vi "create_MagFieldTableObjects.vi"(8 "error in (no error)":errorcluster) -> (0 "error out":errorcluster)   [LabVIEW 2017]
doc: "loads the magfield table data from the MagFieldTables.ini and creates all MagfieldTable objects"
uses:
  Classes/MagFieldTable/MagFieldTable.lvclass
  global variables.vi
  <vilib>/Utility/config.llb/Read Key (String).vi
  Classes/StatusLog/StatusLog.lvclass
  <vilib>/Utility/config.llb/NI_LVConfig.lvlib
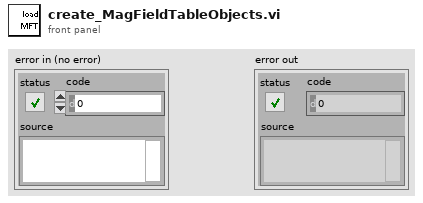
[diagram p1: front panel]
types:
  T1 = typedef "NI_LVConfig.lvlib/Config Data RefNum.ctl" = refnum<k1>
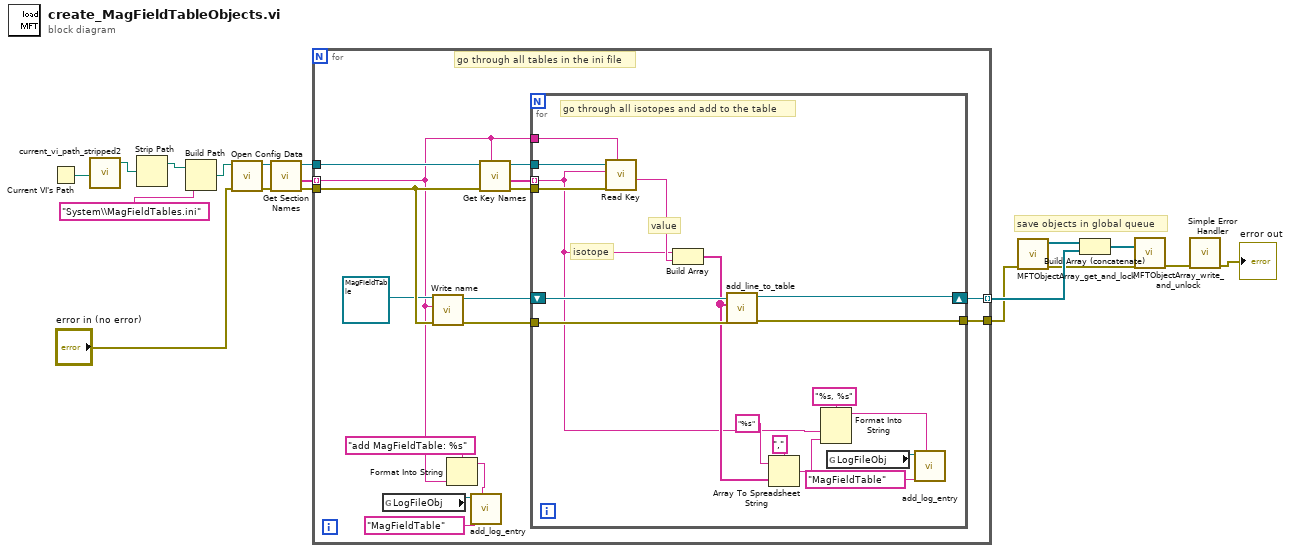
[diagram p0: block diagram]
diagram:
  # "save objects in global queue"
  n1 = Current VI's Path() -> (path=w14:path)
  n2 = call "current_vi_path_stripped2.vi"("current VI Path"=w14) -> ("current VI Path stripped out"=w12:path)  [unwired: 3 in, 1 out]
  n3 = Strip Path(path=w12) -> (stripped path=w13:path)  [unwired: 1 out]
  n4 = Build Path(base path=w13, name or relative path="System\\MagFieldTables.ini") -> (appended path=w15:path)
  n5 = call <vilib>:"Open Config Data.vi"("error in (no error)"="error in (no error)", "configuration file path"=w15) -> ("error out"=w16:errorcluster, "refnum"=w17:T1)  [unwired: 7 in, 1 out]
  n6 = call <vilib>:"Get Section Names.vi"("error in (no error)"=w16, "refnum"=w17) -> ("error out"=w9:errorcluster, "section names"=w11:string[], "refnum out"=w10:T1)  [unwired: 7 in]
  n7 = for {
    tunnel: w11 -> [w20] mode=indexing
    tunnel: w10 -> [w33]
    tunnel: w9 -> [w32]
    tunnel: [w25] -> w5 mode=indexing
    tunnel: [w24] -> w4
    # "go through all tables in the ini file"
    n8 = global read "global variables.vi" "LogFileObj"() -> (w23:refnum<class "StatusLog.lvclass">)
    n9 = call-dynamic "Write name.vi"("error in (no error)"=w32, "name"=w20, "MagFieldTable in"=refnum<class "MagFieldTable.lvclass"> refnum ("MagFieldTable.lvclass")) -> ("error out"=w27:errorcluster, "MagFieldTable out"=w28:refnum<class "MagFieldTable.lvclass">)  [unwired: 7 in]
    n10 = Format Into String(format string="add MagFieldTable: %s", w20) -> (resulting string=w19:string)  [unwired: 2 in, 1 out]
    n11 = call-dynamic "add_log_entry.vi"("new entry"=w19, "log identifiers"="MagFieldTable", "StatusLog in"=w23) -> ()  [unwired: 5 in, 2 out]
    n12 = call <vilib>:"Get Key Names.vi"("section"=w20, "error in (no error)"=w32, "refnum"=w33) -> ("error out"=w30:errorcluster, "key names"=w29:string[], "refnum out"=w31:T1)  [unwired: 5 in, 1 out]
    n13 = for {
      tunnel: w31 -> [w50]
      tunnel: w30 -> [w49]
      tunnel: w29 -> [w35] mode=indexing
      shift-right: [w44] -> w25
      shift-left: w28 -> [w46]
      tunnel: w27 -> [w45]
      tunnel: w20 -> [w48]
      tunnel: [w43] -> w24
      # "value"
      # "isotope"
      # "go through all isotopes and add to the table"
      n14 = call-poly <vilib>:"Read Key.vi"("section"=w48, "error in (no error)"=w49, "key"=w35, "refnum"=w50) -> ("value"=w47:string)  [unwired: 4 in, 3 out]
      n15 = Build Array(w35, w47) -> (w38:string[])
      n16 = call-dynamic "add_line_to_table.vi"("error in (no error)"=w45, "new table line"=w38, "MagFieldTable in"=w46) -> ("error out"=w43:errorcluster, "MagFieldTable out"=w44:refnum<class "MagFieldTable.lvclass">)  [unwired: 7 in]
      n17 = Array To Spreadsheet String(delimiter (Tab)=",", array=w38, 3:"%s" ("format string")) -> (spreadsheet string=w36:string)
      n18 = Format Into String(format string="%s, %s", w35, w36) -> (resulting string=w34:string)  [unwired: 2 in, 1 out]
      n19 = global read "global variables.vi" "LogFileObj"() -> (w42:refnum<class "StatusLog.lvclass">)
      n20 = call-dynamic "add_log_entry.vi"("new entry"=w34, "log identifiers"="MagFieldTable", "StatusLog in"=w42) -> ()  [unwired: 5 in, 2 out]
    }
  }
  n21 = call "MFTObjectArray_get_and_lock.vi"("error in (no error)"=w4) -> ("error out"=w3:errorcluster, "MFTObjects"=w7:refnum<class "MagFieldTable.lvclass">[])  [unwired: 9 in]
  n22 = Build Array (concatenate)(w7, w5) -> (w6:refnum<class "MagFieldTable.lvclass">[])
  n23 = call "MFTObjectArray_write_and_unlock.vi"("error in (no error)"=w3, "MFTObjects"=w6) -> ("error out"=w2:errorcluster)  [unwired: 9 in]
  n24 = call <vilib>:"Simple Error Handler.vi"("error in (no error)"=w2) -> ("error out"=→"error out":errorcluster)  [unwired: 4 in, 4 out]
